vi "Choose Analog Read Mode.vi"(9 "Channel Names":string[](array[string]), 10 "Physical Channels":tag[](array[tag]), 11 "Analog Input Mode":enum16{"High Accuracy", "High Speed"}(ring)) -> (2 "data":waveform(dbl)[](array[waveform]))   [LabVIEW 2020]
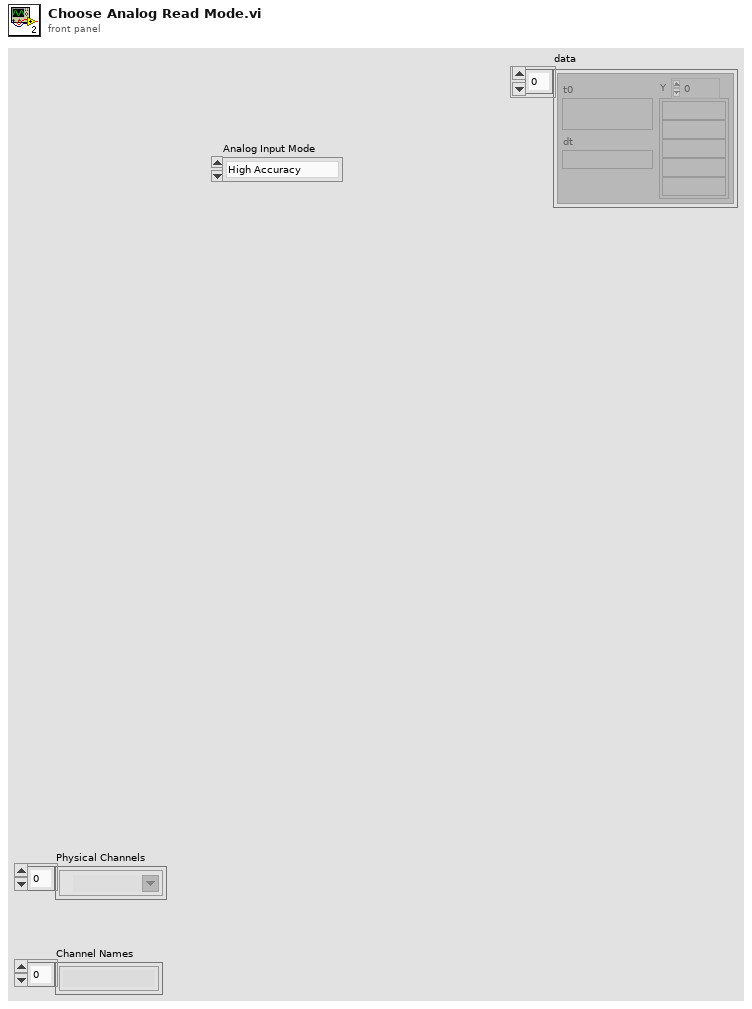
[diagram p1: front panel]
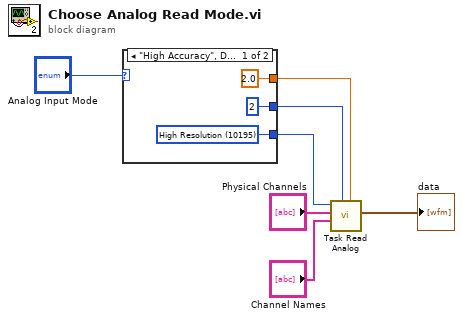
[diagram p0: block diagram]
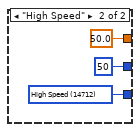
[diagram p2: hidden frame]
diagram:
  n1 = case shown="\"High Accuracy\", Default" "Analog Input Mode" {
    tunnel: [w10 w13] -> w4
    tunnel: [2 ("Samples Per Channel") 50 ("Samples Per Channel")] -> w3
    tunnel: [2.0 ("Sample Rate") 50.0 ("Sample Rate")] -> w2
    frame "High Accuracy", Default {
      w10 = 10195 items=["Automatic"=16097, "High Resolution"=10195, "High Speed"=14712, "Best 50 Hz Rejection"=14713, "Best 60 Hz Rejection"=14714, "Custom"=10137] ("Timing Mode")
    }
    frame "High Speed" {
      w13 = 14712 items=["Automatic"=16097, "High Resolution"=10195, "High Speed"=14712, "Best 50 Hz Rejection"=14713, "Best 60 Hz Rejection"=14714, "Custom"=10137] ("Timing Mode")
    }
  }
  n2 = call "Task Read Analog.vi"("Sample Rate"=w2, "Samples Per Channel"=w3, "Channel Names"="Channel Names", "Physical Channels"="Physical Channels", "Timing Mode"=w4) -> ("data"=→"data":waveform(dbl)[])  [unwired: 4 in, 2 out]
